vi "User Visible Strings.vi"() -> ()   [LabVIEW 2020, in "Text-Based VI Icon.lvlib"]
uses:
  Text-Based VI Icon.lvlib
panel:
  in  "VI Icon Layer Name":string="VI Icon"
  in  "Class Icon Error":string="To set a text icon for this VI, the icon of the class that owns this VI must meet the following requirements:\n\n1. No whitespace at the top of the icon.\n2. The icon is a 32-pixel wide rectangle.\n3. The icon rectangle is at most %d pixels tall.\n\nTo configure a class icon that aligns with these specifications, perform the following steps:\n\n1. Right-click on the respective class and select \"Properties.\"\n2. In the ensuing Properties dialog, click on \"Set Text Icon.\"\n\nUpon successfully assigning a valid class icon, you will then be able to set a text icon for this VI."
  in  "Library Icon Error":string="To set a text icon for this VI, the icon of the library that owns this VI must meet the following requirements:\n\n1. No whitespace at the top of the icon.\n2. The icon is a 32-pixel wide rectangle.\n3. The icon rectangle is at most %d pixels tall.\n\nTo configure a library icon that aligns with these specifications, perform the following steps:\n\n1. Right-click on the respective library and select \"Properties.\"\n2. In the ensuing Properties dialog, click on \"Set Text Icon.\"\n\nUpon successfully assigning a valid library icon, you will then be able to set a text icon for this VI."
  in  "Unsaved VI Error":string="Save the VI before using this function."
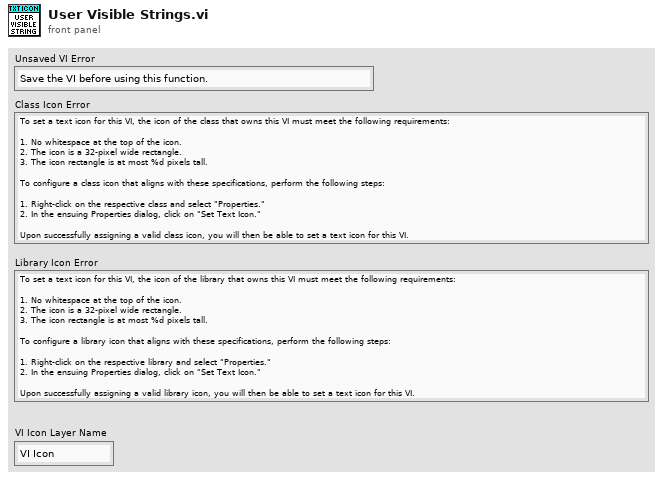
[diagram p1: front panel]
diagram:
